vi "LowPressureVerification.vi"(8 "error in":errorcluster, 11 "S1 in":refnum<class "S1.lvclass">) -> (0 "error out":errorcluster, 3 "S1 out":refnum<class "S1.lvclass">)   [LabVIEW 2018, in "S1.lvclass"]
uses:
  S1.lvclass
  S1.lvclass/S1.ctl
  Public Controls/Outputs.ctl
  Public Controls/ReportHeader.ctl
  IO/IO.lvclass
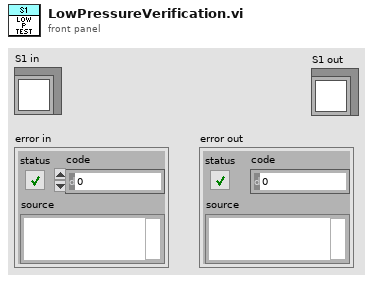
[diagram p1: front panel]
types:
  T1 = typedef "S1.lvclass/Outputs.ctl" = cluster{"LoP":bool, "HiP":bool, "Z1Vent":bool, "Z2Vent":bool, "Z3Vent":bool, "IsLidLock":bool}
  T2 = typedef "S1.lvclass/ReportHeader.ctl" = string
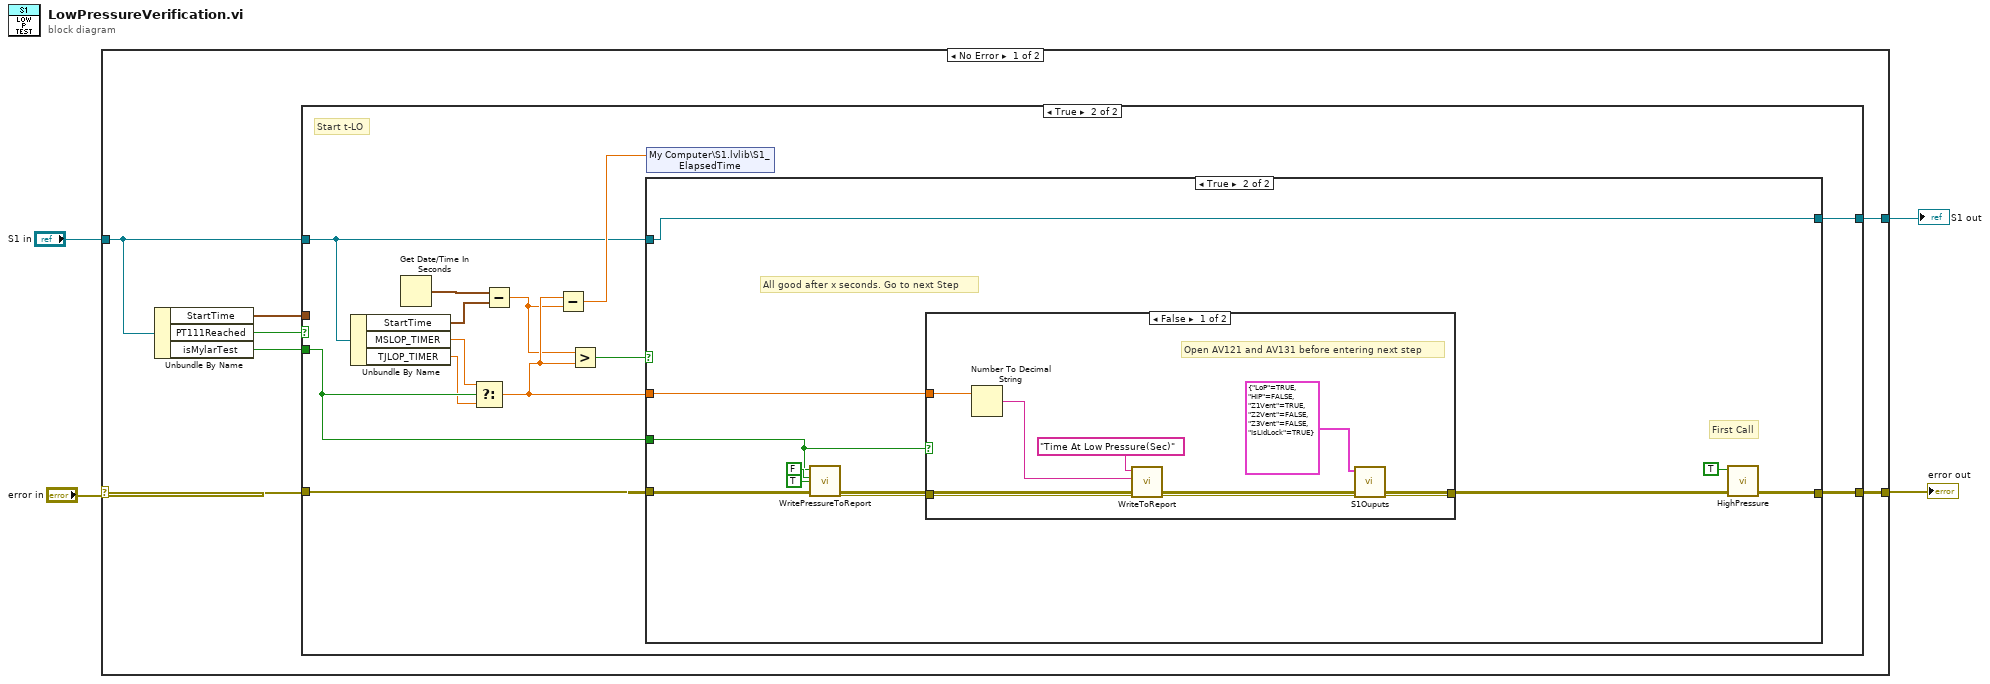
[diagram p0: block diagram]
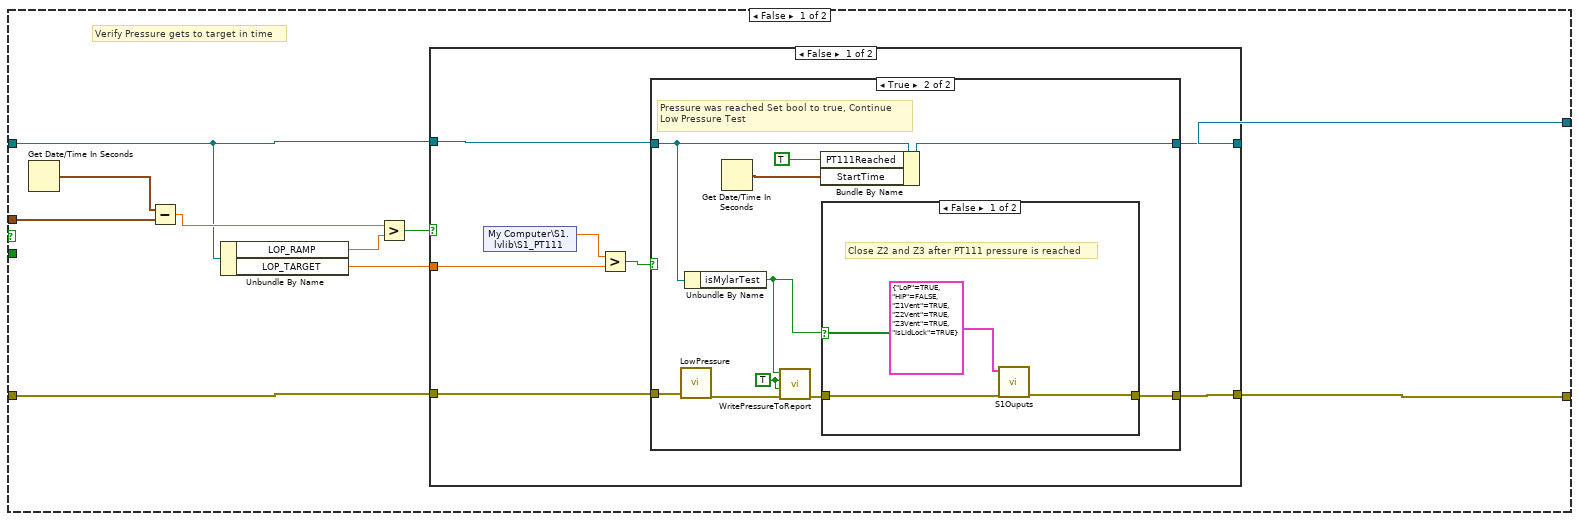
[diagram p2: hidden frame]
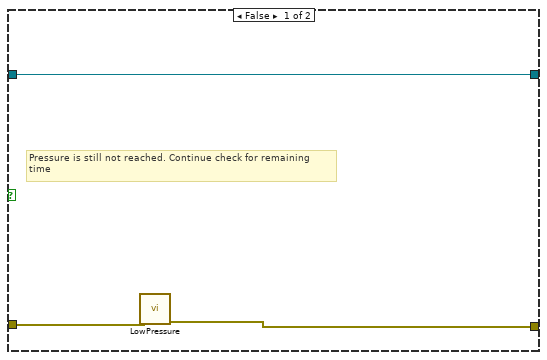
[diagram p3: hidden frame]
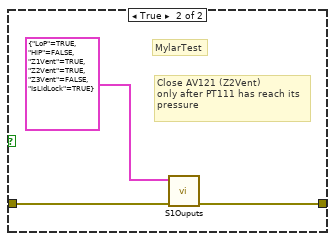
[diagram p4: hidden frame]
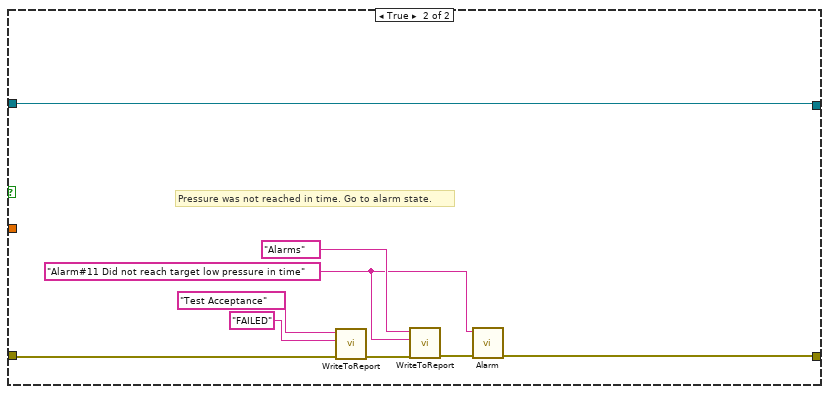
[diagram p5: hidden frame]
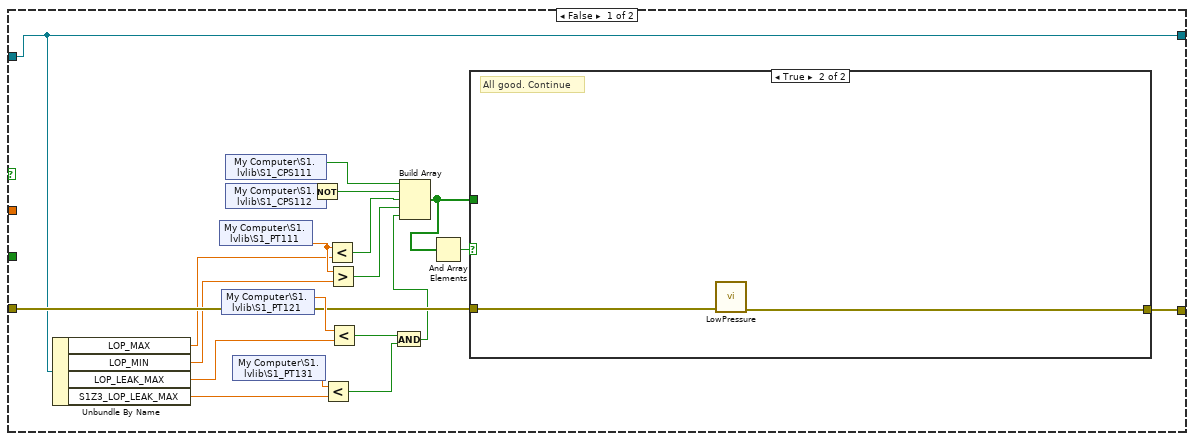
[diagram p6: hidden frame]
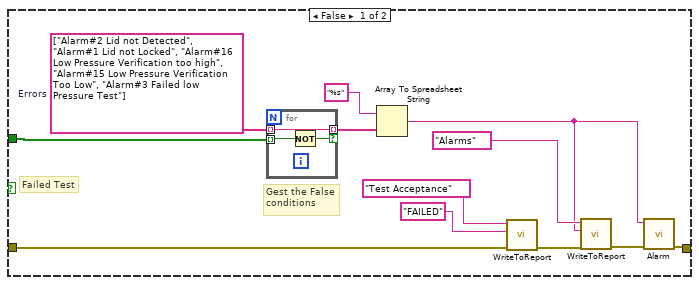
[diagram p7: hidden frame]
diagram:
  n1 = case shown="No Error" "error in" {
    selector: "error in" -> [w11 w127]
    tunnel: [w7 w127] -> w4
    tunnel: "S1 in" -> [w6 w126]
    tunnel: [w8 w126] -> w1
    frame No Error {
      n2 = Unbundle By Name(w6) -> ("StartTime"=w9:timestamp, "PT111Reached"=w10:bool, "isMylarTest"=w5:bool)
      n3 = case shown="True" w10 {
        tunnel: w11 -> [w18 w69]
        tunnel: [w16 w65] -> w7
        tunnel: w9 -> [w20 _]
        tunnel: w6 -> [w14 w60]
        tunnel: [w15 w59] -> w8
        tunnel: w5 -> [_ w64]
        frame False {
          # "Verify Pressure gets to target in time"
          n4 = Get Date/Time In Seconds() -> (seconds since 1Jan1904=w21:timestamp)
          n5 = Subtract(x=w21, y=w20) -> (x-y=w19:dbl)
          n6 = Unbundle By Name(w14) -> ("LOP_RAMP"=w13:dbl, "LOP_TARGET"=w12:dbl)
          n7 = Greater?(x=w19, y=w13) -> (0:w17:bool)
          n8 = case shown="False" w17 {
            tunnel: w18 -> [w24 w51]
            tunnel: [w23 w53] -> w16
            tunnel: w14 -> [w26 w50]
            tunnel: [w25 w50] -> w15
            tunnel: w12 -> [w22 _]
            frame False {
              n9 = shared-variable "My Computer\\S1.lvlib\\S1_PT111"() -> (w28:dbl)  [unwired: 1 in, 1 out]
              n10 = Greater?(x=w28, y=w22) -> (0:w27:bool)
              n11 = case shown="True" w27 {
                tunnel: w26 -> [w30 w38]
                tunnel: [w30 w41] -> w25
                tunnel: w24 -> [w29 w37]
                tunnel: [w31 w36] -> w23
                frame False {
                  # "Pressure is still not reached. Continue check for remaining\ntime"
                  n12 = call "LowPressure.vi"("error in"=w29) -> ("error out"=w31:errorcluster)  [unwired: 10 in]
                }
                frame True {
                  w35 = TRUE ("Initial")
                  # "Pressure was reached Set bool to true, Continue\nLow Pressure Test"
                  n13 = call "LowPressure.vi"("error in"=w37) -> ("error out"=w33:errorcluster)  [unwired: 10 in]
                  n14 = Unbundle By Name(w38) -> ("isMylarTest"=w34:bool)
                  n15 = Get Date/Time In Seconds() -> (seconds since 1Jan1904=w39:timestamp)
                  n16 = call "WritePressureToReport.vi"("error in (no error)"=w33, "LowPressure"=w35, "Initial"=w35, "isMylarTest"=w34) -> ("error out"=w32:errorcluster)  [unwired: 7 in]
                  n17 = Bundle By Name(cluster=w38, "PT111Reached"=TRUE ("PT111ReachedPressure"), "StartTime"=w39) -> (w41:refnum<class "S1.lvclass">)
                  n18 = case shown="False" w34 {
                    tunnel: w32 -> [w44 w45]
                    tunnel: [w42 w46] -> w36
                    frame False {
                      # "Close Z2 and Z3 after PT111 pressure is reached"
                      n19 = call "S1Ouputs.vi"("error in"=w44, "SIOutputs"=T1 {"LoP"=TRUE, "HiP"=FALSE, "Z1Vent"=TRUE, "Z2Vent"=TRUE, "Z3Vent"=TRUE, "IsLidLock"=TRUE}) -> ("error out"=w42:errorcluster)  [unwired: 9 in]
                    }
                    frame True {
                      # "MylarTest"
                      # "Close AV121 (Z2Vent)\nonly after PT111 has reach its\npressure"
                      n20 = call "S1Ouputs.vi"("error in"=w45, "SIOutputs"=T1 {"LoP"=TRUE, "HiP"=FALSE, "Z1Vent"=TRUE, "Z2Vent"=TRUE, "Z3Vent"=FALSE, "IsLidLock"=TRUE}) -> ("error out"=w46:errorcluster)  [unwired: 9 in]
                    }
                  }
                }
              }
            }
            frame True {
              w49 = "Alarm#11 Did not reach target low pressure in time" ("Value")
              # "Pressure was not reached in time. Go to alarm state."
              n21 = call "WriteToReport.vi"("error in"=w51, "Value"="FAILED", "Header"=T2 "Test Acceptance") -> ("error out"=w56:errorcluster)  [unwired: 8 in]
              n22 = call "WriteToReport.vi"("error in"=w56, "Value"=w49, "Header"="Alarms") -> ("error out"=w54:errorcluster)  [unwired: 8 in]
              n23 = call "Alarm.vi"("error in"=w54, "Alarm"=w49) -> ("error out"=w53:errorcluster)  [unwired: 9 in]
            }
          }
        }
        frame True {
          # "Start t-LO"
          n24 = Unbundle By Name(w60) -> ("StartTime"=w67:timestamp, "MSLOP_TIMER"=w63:dbl, "TJLOP_TIMER"=w62:dbl)
          n25 = Get Date/Time In Seconds() -> (seconds since 1Jan1904=w68:timestamp)
          n26 = Select(t=w63, s=w64, f=w62) -> (s? t:f=w58:dbl)
          n27 = Subtract(x=w68, y=w67) -> (x-y=w57:dbl)
          n28 = Subtract(x=w58, y=w57) -> (x-y=w61:dbl)
          n29 = Greater?(x=w57, y=w58) -> (0:w66:bool)
          n30 = case shown="True" w66 {
            tunnel: w69 -> [w90 w113]
            tunnel: [w87 w117] -> w65
            tunnel: w64 -> [_ w110]
            tunnel: w58 -> [_ w109]
            tunnel: w60 -> [w74 w108]
            tunnel: [w74 w108] -> w59
            frame False {
              n31 = Unbundle By Name(w74) -> ("LOP_MAX"=w71:dbl, "LOP_MIN"=w70:dbl, "LOP_LEAK_MAX"=w73:dbl, "S1Z3_LOP_LEAK_MAX"=w72:dbl)
              n32 = shared-variable "My Computer\\S1.lvlib\\S1_PT111"() -> (w86:dbl)  [unwired: 1 in, 1 out]
              n33 = shared-variable "My Computer\\S1.lvlib\\S1_PT121"(error in=w90) -> (w89:dbl, error out=w88:errorcluster)
              n34 = shared-variable "My Computer\\S1.lvlib\\S1_CPS111"() -> (w81:bool)  [unwired: 1 in, 1 out]
              n35 = shared-variable "My Computer\\S1.lvlib\\S1_CPS112"() -> (w80:bool)  [unwired: 1 in, 1 out]
              n36 = shared-variable "My Computer\\S1.lvlib\\S1_PT131"() -> (w76:dbl)  [unwired: 1 in, 1 out]
              n37 = Not(x=w80) -> (.not. x?=w75:bool)
              n38 = Less?(x=w76, y=w72) -> (x < y?=w78:bool)
              n39 = Less?(x=w86, y=w71) -> (x < y?=w85:bool)
              n40 = Greater?(x=w86, y=w70) -> (0:w84:bool)
              n41 = Less?(x=w89, y=w73) -> (x < y?=w79:bool)
              n42 = And(x=w79, y=w78) -> (x .and. y?=w77:bool)
              n43 = Build Array(w81, w75, w85, w84, w77) -> (w82:bool[])
              n44 = And Array Elements(Boolean array=w82) -> (logical AND=w83:bool)
              n45 = case shown="True" w83 {
                tunnel: w88 -> [w97 w107]
                tunnel: [w99 w106] -> w87
                tunnel: w82 -> [w96 _]
                frame False {
                  w95 = string[] ["Alarm#2 Lid not Detected", "Alarm#1 Lid not Locked", "Alarm#16 Low Pressure Verification too high", "Alarm#15 Low Pressure Verification Too Low", "Alarm#3 Failed low Pressure Test"]  # Errors
                  # "Failed Test"
                  # "Gest the False\nconditions"
                  n46 = for {
                    tunnel: w96 -> [w104] mode=indexing
                    tunnel: w95 -> [w105] mode=indexing
                    tunnel: [w105] -> w94 mode=indexing if=w103
                    n47 = Not(x=w104) -> (.not. x?=w103:bool)
                  }
                  n48 = Array To Spreadsheet String(array=w94, 3:"%s" ("format string")) -> (spreadsheet string=w92:string)  [unwired: 1 in]
                  n49 = call "WriteToReport.vi"("error in"=w97, "Value"="FAILED", "Header"=T2 "Test Acceptance") -> ("error out"=w102:errorcluster)  [unwired: 8 in]
                  n50 = call "WriteToReport.vi"("error in"=w102, "Value"=w92, "Header"="Alarms") -> ("error out"=w100:errorcluster)  [unwired: 8 in]
                  n51 = call "Alarm.vi"("error in"=w100, "Alarm"=w92) -> ("error out"=w99:errorcluster)  [unwired: 9 in]
                }
                frame True {
                  # "All good. Continue"
                  n52 = call "LowPressure.vi"("error in"=w107) -> ("error out"=w106:errorcluster)  [unwired: 10 in]
                }
              }
            }
            frame True {
              # "First Call"
              # "All good after x seconds. Go to next Step"
              n53 = call "WritePressureToReport.vi"("error in (no error)"=w113, "LowPressure"=TRUE, "Initial"=FALSE, "isMylarTest"=w110) -> ("error out"=w112:errorcluster)  [unwired: 7 in]
              n54 = case shown="False" w110 {
                tunnel: w112 -> [w124 w125]
                tunnel: [w118 w125] -> w111
                tunnel: w109 -> [w121 _]
                frame False {
                  # "Open AV121 and AV131 before entering next step"
                  n55 = Number To Decimal String(number=w121) -> (decimal integer string=w123:string)  [unwired: 1 in]
                  n56 = call "WriteToReport.vi"("error in"=w124, "Value"=w123, "Header"="Time At Low Pressure(Sec)" ("decimal integer string")) -> ("error out"=w119:errorcluster)  [unwired: 8 in]
                  n57 = call "S1Ouputs.vi"("error in"=w119, "SIOutputs"=T1 {"LoP"=TRUE, "HiP"=FALSE, "Z1Vent"=TRUE, "Z2Vent"=FALSE, "Z3Vent"=FALSE, "IsLidLock"=TRUE}) -> ("error out"=w118:errorcluster)  [unwired: 9 in]
                }
                frame True {
                }
              }
              n58 = call "HighPressure.vi"("error in"=w111, "FirstCall(F)"=TRUE) -> ("error out"=w117:errorcluster)  [unwired: 9 in]
            }
          }
          n59 = shared-variable "My Computer\\S1.lvlib\\S1_ElapsedTime"(w61) -> ()  [unwired: 1 in, 1 out]
        }
      }
    }
    frame Error {
    }
  }
  "error out" <- w4
  "S1 out" <- w1
